vi "filterNumberOfRobots.vi"(8 "error in (no error)":errorcluster, 9 "Game":refnum<class "Game.lvclass">, 10 "previousNumberOfRobots":i32, 11 "MarkerSkill in":refnum<class "MarkerSkill.lvclass">) -> (0 "error out":errorcluster, 2 "finalNumberOfRobots":i32, 3 "MarkerSkill out":refnum<class "MarkerSkill.lvclass">)   [LabVIEW 2020, in "MarkerSkill.lvclass"]
uses:
  MarkerSkill.lvclass
  Game_class/Game.lvclass
  Game_class/Game.lvclass/Game.ctl
  Team_class/Team.lvclass/Team.ctl
  Game_class/Read AllyRef.vi
  Team_class/Read RobotRef.vi
  Ally_class/Ally.lvclass
  C:/Users/anton/Desktop/RoboIME/SSL_COMP/SSL_AI/Team_class/Team.lvclass
  Robot_class/Robot.lvclass
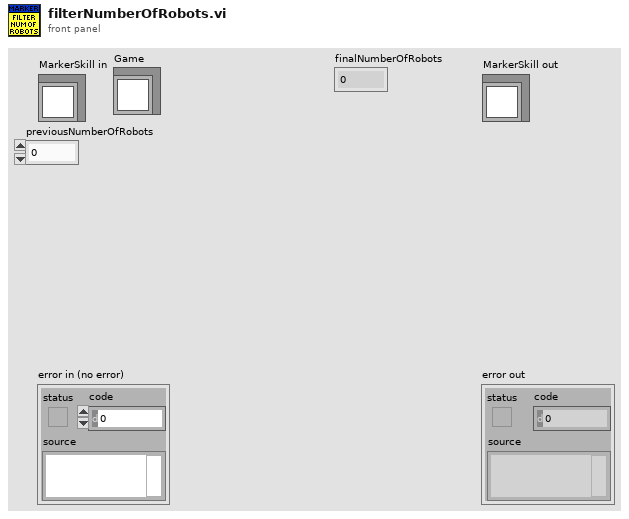
[diagram p1: front panel]
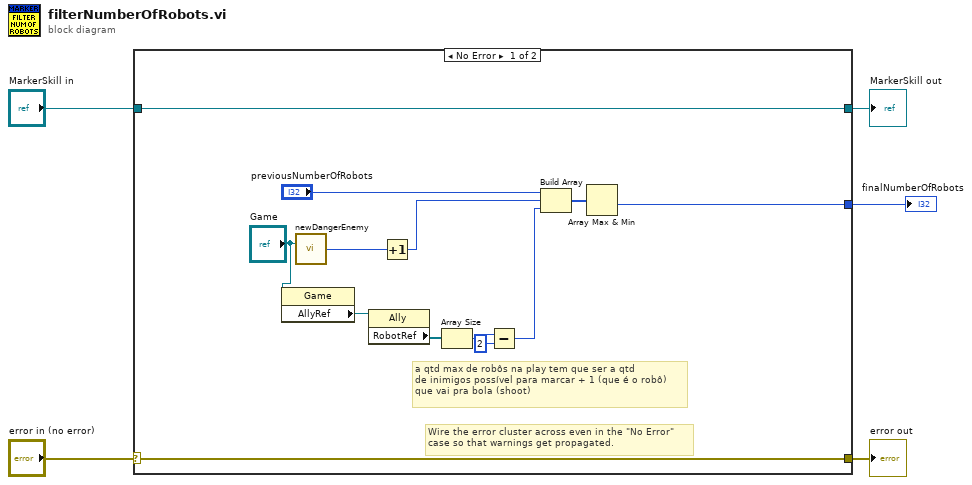
[diagram p0: block diagram]
diagram:
  n1 = case shown="No Error" "error in (no error)" {
    selector: "error in (no error)" -> [w17 w20]
    tunnel: [w17 w20] -> w4
    tunnel: [w18 w19] -> w2
    tunnel: "MarkerSkill in" -> [w18 w19]
    tunnel: [w12 _] -> w1
    frame No Error {
      # "a qtd max de robôs na play tem que ser a qtd\nde inimigos possível para marcar + 1 (que é o robô)\nque vai pra bola (shoot)"
      # "Wire the error cluster across even in the \"No Error\"\ncase so that warnings get propagated."
      n2 = property class="Game"(reference="Game") -> ("AllyRef"=w10:refnum<class "Ally.lvclass">)  [unwired: 1 in, 2 out]
      n3 = call "newDangerEnemy.vi"("Game"="Game") -> ("numberOfPossible\nEnemiesToMark"=w14:i32)  [unwired: 11 in, 3 out]
      n4 = property class="Ally"(reference=w10) -> ("RobotRef"=w9:refnum<class "Robot.lvclass">[])  [unwired: 1 in, 2 out]
      n5 = Increment(x=w14) -> (x+1=w16:i32)
      n6 = Array Size(array=w9) -> (size(s)=w8:i32)
      n7 = Subtract(x=w8, y=2) -> (x-y=w6:i32)
      n8 = Build Array("previousNumberOfRobots", w16, w6) -> (w15:i32[])
      n9 = Array Max & Min(array=w15) -> (min value=w12:i32)  [unwired: 3 out]
    }
    frame Error {
    }
  }
  "error out" <- w4
  "MarkerSkill out" <- w2
  "finalNumberOfRobots" <- w1
